vi "gui_control.vi"() -> ()   [LabVIEW 2020]
uses:
  <vilib>/Instr/_visa.llb/VISA Configure Serial Port (Instr).vi
panel:
  out "Response":string
  in  "CONNECTION":bool
  out "Bytes Read":u32
  in  "VISA Resource":refnum<visa-resource-name>="COM1"
  in  "Tab Control":enum32{"Page 1", "Page 2"}(tab)
  in  "End":timestamp caption="Day End" format="%<%H:%M>T"
  in  "Start":timestamp caption="Day Start" format="%<%H:%M>T"
  in  "SEND LED":bool caption="Boolean"
  out "Color Box":u32(colorbox)
  in  "R":u8
  in  "G":u8
  in  "B":u8
  in  "SEND RTC":bool caption="Boolean"
  in  "SEND INT":bool caption="Boolean"
  in  "INT 2":u8 caption="Brightness"
  in  "B 2":u8 caption="B"
  in  "G 2":u8 caption="G"
  in  "R 2":u8 caption="R"
  out "Color Box 2":u32(colorbox)
  in  "SEND RTC 2":bool caption="Boolean"
  in  "SEND LED 2":bool caption="Boolean"
  in  "End 2":timestamp caption="Day End" format="%<%H:%M>T"
  in  "Start 2":timestamp caption="Day Start" format="%<%H:%M>T"
  in  "SEND INT 2":bool caption="Boolean"
  in  "INT":u8 caption="Brightness"
  # "Serial Monitor"
  # "--- Box 0 ---"
  # "Auto LED Timer"
  # "Manual Color Control"
  # "--- Box 1 ---"
  # "Auto LED Timer"
  # "Manual Color Control"
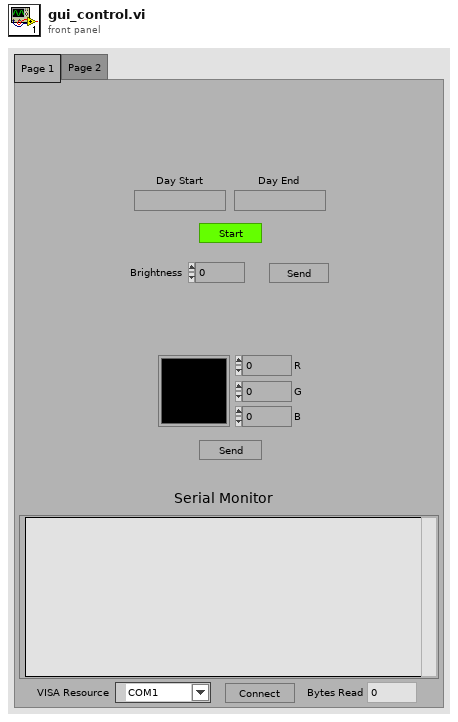
[diagram p1: front panel]
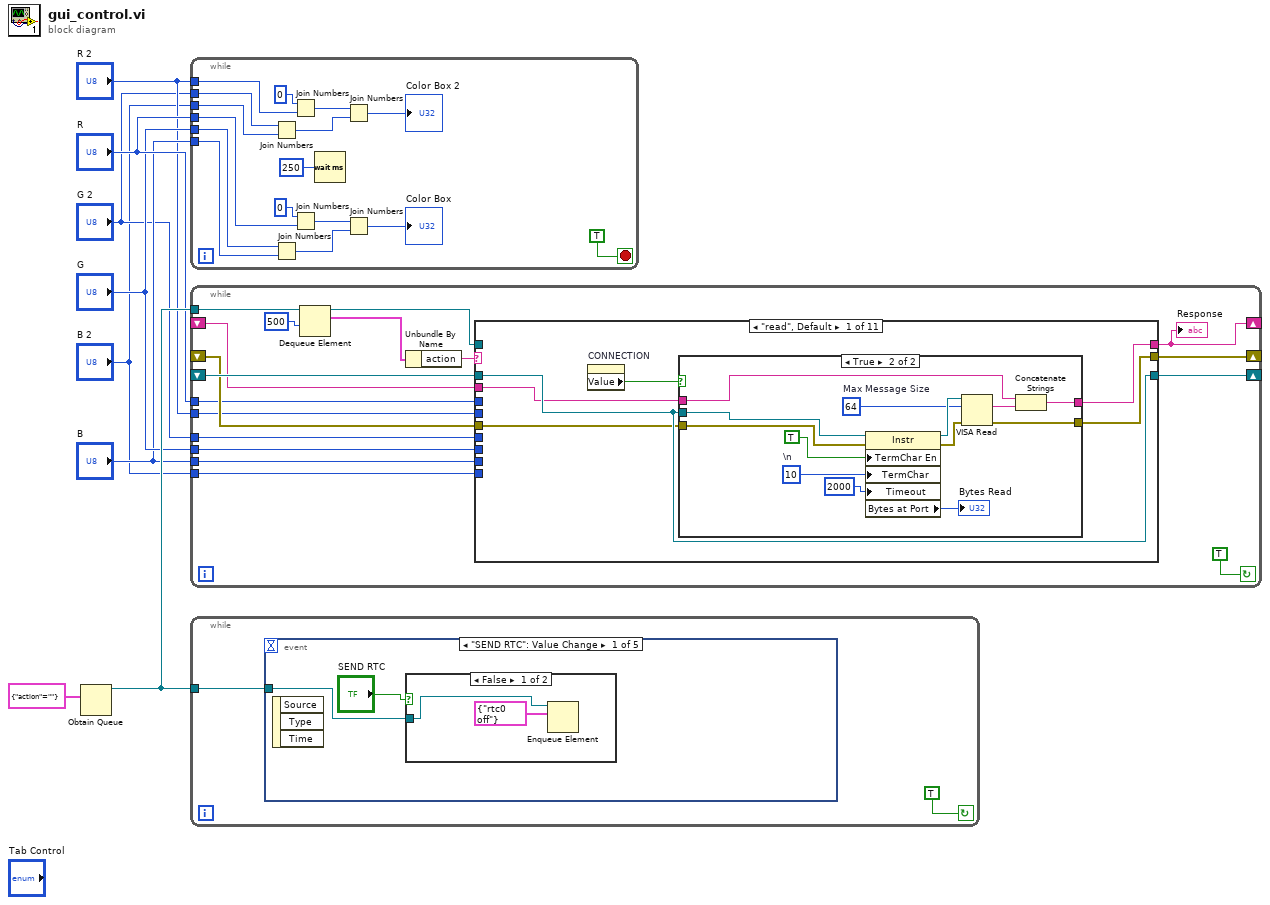
[diagram p0: block diagram]
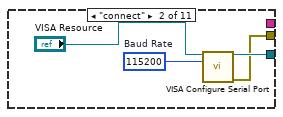
[diagram p3: hidden frame]
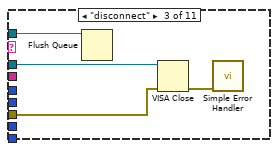
[diagram p4: hidden frame]
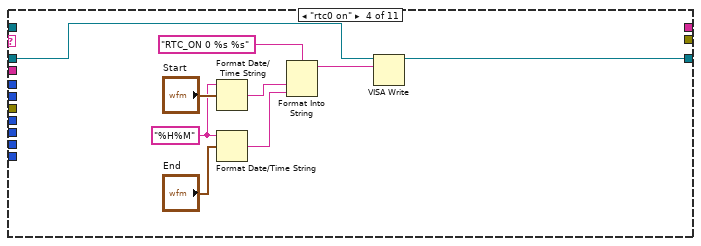
[diagram p5: hidden frame]
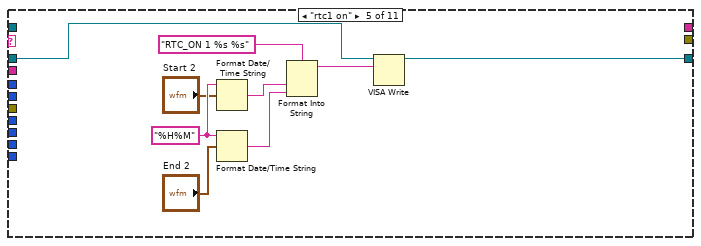
[diagram p6: hidden frame]
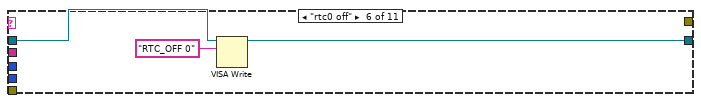
[diagram p7: hidden frame]
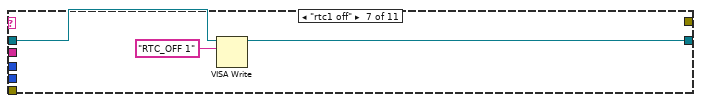
[diagram p8: hidden frame]
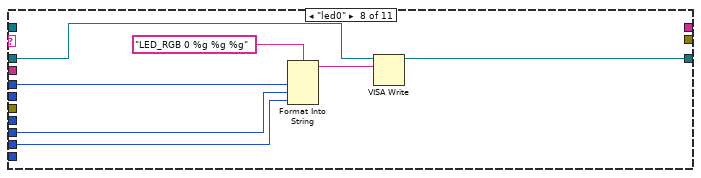
[diagram p9: hidden frame]
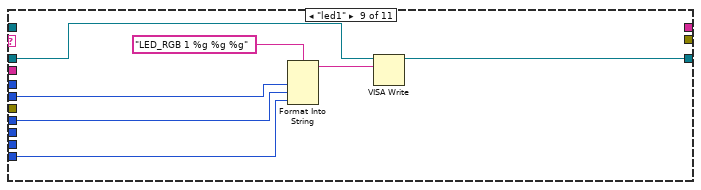
[diagram p10: hidden frame]
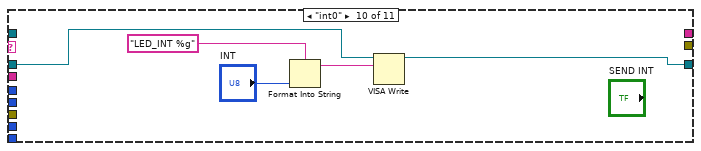
[diagram p11: hidden frame]
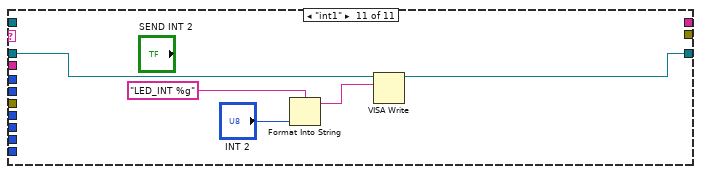
[diagram p12: hidden frame]
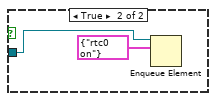
[diagram p13: hidden frame]
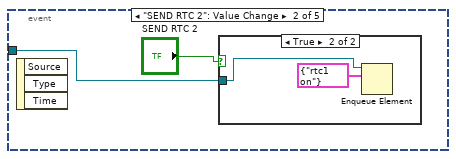
[diagram p14: hidden frame]
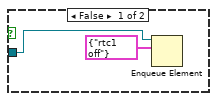
[diagram p15: hidden frame]
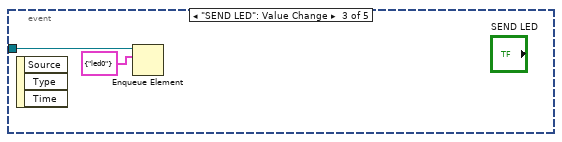
[diagram p16: hidden frame]
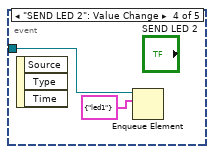
[diagram p17: hidden frame]
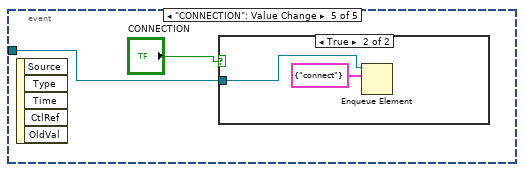
[diagram p18: hidden frame]
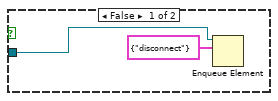
[diagram p19: hidden frame]
diagram:
  n1 = Obtain Queue(element data type=cluster{"action":string} {"action"=""}) -> (queue out=w7:refnum<queue>)  [unwired: 4 in, 2 out]
  n2 = while {
    tunnel: "R" -> [w18]
    tunnel: "G" -> [w17]
    tunnel: "B" -> [w16]
    tunnel: "R 2" -> [w14]
    tunnel: "G 2" -> [w12]
    tunnel: "B 2" -> [w11]
    stop <- TRUE stop-if-true
    n3 = Join Numbers(hi=w12, lo=w11) -> ((hi.lo)=w10:u16)
    n4 = Join Numbers(hi=w17, lo=w16) -> ((hi.lo)=w20:u16)
    n5 = Join Numbers(hi=u8 0, lo=w14) -> ((hi.lo)=w9:u16)
    n6 = Join Numbers(hi=u8 0, lo=w18) -> ((hi.lo)=w21:u16)
    n7 = Wait (ms)(milliseconds to wait=u32 250) -> ()  [unwired: 1 out]
    n8 = Join Numbers(hi=w9, lo=w10) -> ((hi.lo)=→"Color Box 2":u32)
    n9 = Join Numbers(hi=w21, lo=w20) -> ((hi.lo)=→"Color Box":u32)
  }
  n10 = while {
    tunnel: w7 -> [w42]
    shift-right: [w37] -> _
    shift-left: _ -> [w36]
    shift-right: [w35] -> _
    shift-left: _ -> [w34]
    tunnel: "R" -> [w33]
    tunnel: "G" -> [w32]
    tunnel: "B" -> [w31]
    tunnel: "R 2" -> [w30]
    tunnel: "G 2" -> [w29]
    tunnel: "B 2" -> [w28]
    shift-right: [w26] -> _
    shift-left: _ -> [w27]
    stop <- TRUE continue-if-true
    n11 = Dequeue Element(queue=w42, timeout in ms (-1)=500) -> (queue out=w38:refnum<queue>, element=w40:cluster{"action":string})  [unwired: 1 in, 2 out]
    n12 = Unbundle By Name(w40) -> ("action"=w39:string)
    n13 = case shown="\"read\", Default" w39 {
      tunnel: w38 -> [_ _ w66 _ _ _ _ _ _ _ _]
      tunnel: [w48 w63 _ w70 w80 w89 w91 w97 w104 w108 w114] -> w37
      tunnel: w36 -> [w48 _ w69 w71 w79 w90 w92 w98 w105 w109 w115]
      tunnel: [w46 w62 _ _ _ _ _ _ _ _ _] -> w35
      tunnel: w34 -> [w47 _ w67 _ _ _ _ _ _ _ _]
      tunnel: w33 -> [_ _ _ _ _ _ _ w96 _ _ _]
      tunnel: w32 -> [_ _ _ _ _ _ _ w95 _ _ _]
      tunnel: w31 -> [_ _ _ _ _ _ _ w94 _ _ _]
      tunnel: w30 -> [_ _ _ _ _ _ _ _ w103 _ _]
      tunnel: w29 -> [_ _ _ _ _ _ _ _ w102 _ _]
      tunnel: w28 -> [_ _ _ _ _ _ _ _ w101 _ _]
      tunnel: [w44 _ _ _ _ _ _ _ _ _ _] -> w26
      tunnel: w27 -> [w45 _ _ _ _ _ _ _ _ _ _]
      frame "read", Default {
        n14 = property on="CONNECTION" class="Bool (strict)"() -> ("Value"=w43:bool)  [unwired: 2 in, 2 out]
        n15 = case shown="True" w43 {
          tunnel: w48 -> [_ w54]
          tunnel: w47 -> [_ w53]
          tunnel: [_ w52] -> w46
          tunnel: w45 -> [_ w51]
          tunnel: [_ w49] -> w44
          frame False {
          }
          frame True {
            w58 = u32 64  # Max Message Size
            w56 = u8 10  # \n
            n16 = property class="Instr"(reference=w54, error in=w53, "TermChar En"=TRUE ("Message Based Settings:Termination Character Enable"), "TermChar"=w56, "Timeout"=u32 2000 ("General Settings:Timeout Value")) -> (reference out=w61:refnum<visa-resource-name>, error out=w60:errorcluster, "Bytes at Port"=→"Bytes Read":u32)
            n17 = VISA Read(VISA resource name=w61, byte count=w58, error in (no error)=w60) -> (read buffer=w50:string, error out=w52:errorcluster)  [unwired: 2 out]
            n18 = Concatenate Strings(w51, w50) -> (w49:string)
          }
        }
      }
      frame "connect" {
        w64 = u32 115200  # Baud Rate
        n19 = call-poly "VISA Configure Serial Port"("VISA resource name"="VISA Resource", "baud rate (9600)"=w64) -> ("VISA resource name out"=w63:refnum<visa-resource-name>, "error out"=w62:errorcluster)  [unwired: 7 in, 5 out]
      }
      frame "disconnect" {
        n20 = Flush Queue(queue=w66) -> ()  [unwired: 1 in, 3 out]
        n21 = VISA Close(VISA resource name=w69, error in (no error)=w67) -> (error out=w68:errorcluster)
        n22 = call <vilib>:"Simple Error Handler.vi"("error in (no error)"=w68) -> ()  [unwired: 1 in, 8 out]
      }
      frame "rtc0 on" {
        w72 = "%H%M"
        n23 = Format Date/Time String(time format string (%c)=w72, seconds (now)="Start") -> (date/time string=w78:string)  [unwired: 1 in]
        n24 = Format Date/Time String(time format string (%c)=w72, seconds (now)="End") -> (date/time string=w77:string)  [unwired: 1 in]
        n25 = Format Into String(format string="RTC_ON 0 %s %s", w78, w77) -> (resulting string=w74:string)  [unwired: 2 in, 1 out]
        n26 = VISA Write(VISA resource name=w71, write buffer=w74) -> (VISA resource name out=w70:refnum<visa-resource-name>)  [unwired: 1 in, 2 out]
      }
      frame "rtc1 on" {
        w85 = "%H%M"
        n27 = Format Date/Time String(time format string (%c)=w85, seconds (now)="Start 2") -> (date/time string=w83:string)  [unwired: 1 in]
        n28 = Format Date/Time String(time format string (%c)=w85, seconds (now)="End 2") -> (date/time string=w84:string)  [unwired: 1 in]
        n29 = Format Into String(format string="RTC_ON 1 %s %s", w83, w84) -> (resulting string=w86:string)  [unwired: 2 in, 1 out]
        n30 = VISA Write(VISA resource name=w79, write buffer=w86) -> (VISA resource name out=w80:refnum<visa-resource-name>)  [unwired: 1 in, 2 out]
      }
      frame "rtc0 off" {
        n31 = VISA Write(VISA resource name=w90, write buffer="RTC_OFF 0" ("format string")) -> (VISA resource name out=w89:refnum<visa-resource-name>)  [unwired: 1 in, 2 out]
      }
      frame "rtc1 off" {
        n32 = VISA Write(VISA resource name=w92, write buffer="RTC_OFF 1" ("format string")) -> (VISA resource name out=w91:refnum<visa-resource-name>)  [unwired: 1 in, 2 out]
      }
      frame "led0" {
        n33 = Format Into String(format string="LED_RGB 0 %g %g %g", w96, w95, w94) -> (resulting string=w99:string)  [unwired: 2 in, 1 out]
        n34 = VISA Write(VISA resource name=w98, write buffer=w99) -> (VISA resource name out=w97:refnum<visa-resource-name>)  [unwired: 1 in, 2 out]
      }
      frame "led1" {
        n35 = Format Into String(format string="LED_RGB 1 %g %g %g", w103, w102, w101) -> (resulting string=w106:string)  [unwired: 2 in, 1 out]
        n36 = VISA Write(VISA resource name=w105, write buffer=w106) -> (VISA resource name out=w104:refnum<visa-resource-name>)  [unwired: 1 in, 2 out]
      }
      frame "int0" {
        n37 = Format Into String(format string="LED_INT %g", "INT") -> (resulting string=w110:string)  [unwired: 2 in, 1 out]
        n38 = VISA Write(VISA resource name=w109, write buffer=w110) -> (VISA resource name out=w108:refnum<visa-resource-name>)  [unwired: 1 in, 2 out]
      }
      frame "int1" {
        n39 = Format Into String(format string="LED_INT %g", "INT 2") -> (resulting string=w116:string)  [unwired: 2 in, 1 out]
        n40 = VISA Write(VISA resource name=w115, write buffer=w116) -> (VISA resource name out=w114:refnum<visa-resource-name>)  [unwired: 1 in, 2 out]
      }
    }
    "Response" <- w26
  }
  n41 = while {
    tunnel: w7 -> [w119]
    stop <- TRUE continue-if-true
    n42 = event shown="[0] \"SEND RTC\": Value Change" {
      selector: _ -> [_ _ _ _ _]
      dyn-events: _ -> [_ _ _ _ _]
      timeout: _ -> [_ _ _ _ _]
      tunnel: w119 -> [w120 w126 w132 w134 w137]
      event "SEND RTC": Value Change {
        n43 = event-data() -> ()  [unwired: 1 in, 3 out]
        n44 = case shown="False" "SEND RTC" {
          tunnel: w120 -> [w122 w124]
          frame False {
            n45 = Enqueue Element(queue=w122, element=cluster{"action":string} {"action"="rtc0 off"}) -> ()  [unwired: 2 in, 3 out]
          }
          frame True {
            n46 = Enqueue Element(queue=w124, element=cluster{"action":string} {"action"="rtc0 on"}) -> ()  [unwired: 2 in, 3 out]
          }
        }
      }
      event "SEND RTC 2": Value Change {
        n47 = event-data() -> ()  [unwired: 1 in, 3 out]
        n48 = case shown="True" "SEND RTC 2" {
          tunnel: w126 -> [w128 w130]
          frame False {
            n49 = Enqueue Element(queue=w128, element=cluster{"action":string} {"action"="rtc1 off"}) -> ()  [unwired: 2 in, 3 out]
          }
          frame True {
            n50 = Enqueue Element(queue=w130, element=cluster{"action":string} {"action"="rtc1 on"}) -> ()  [unwired: 2 in, 3 out]
          }
        }
      }
      event "SEND LED": Value Change {
        n51 = event-data() -> ()  [unwired: 1 in, 3 out]
        n52 = Enqueue Element(queue=w132, element=cluster{"action":string} {"action"="led0"}) -> ()  [unwired: 2 in, 3 out]
      }
      event "SEND LED 2": Value Change {
        n53 = event-data() -> ()  [unwired: 1 in, 3 out]
        n54 = Enqueue Element(queue=w134, element=cluster{"action":string} {"action"="led1"}) -> ()  [unwired: 2 in, 3 out]
      }
      event "CONNECTION": Value Change {
        n55 = event-data() -> ()  [unwired: 1 in, 5 out]
        n56 = case shown="True" "CONNECTION" {
          tunnel: w137 -> [w138 w141]
          frame False {
            n57 = Enqueue Element(queue=w138, element=cluster{"action":string} {"action"="disconnect"}) -> ()  [unwired: 2 in, 3 out]
          }
          frame True {
            n58 = Enqueue Element(queue=w141, element=cluster{"action":string} {"action"="connect"}) -> ()  [unwired: 2 in, 3 out]
          }
        }
      }
    }
  }
